vi "Get_SA_Spectrum_SubVI.vi"(8 "error in (no error)":errorcluster, 11 "IVI Refnum in":refnum<k15>) -> (0 "error out":errorcluster, 3 "IVI Refnum out":refnum<k15>)   [LabVIEW 2023]
uses:
  <instrlib>/Keysight XSAn/Keysight XSAn.lvlib
panel:
  out "Spectrum":cluster{"Frequency":dbl[], "Amplitude":dbl[]}
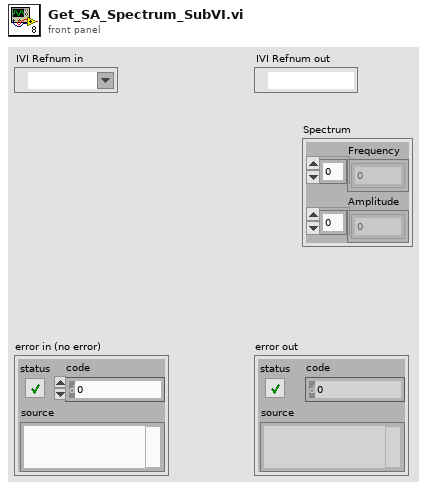
[diagram p1: front panel]
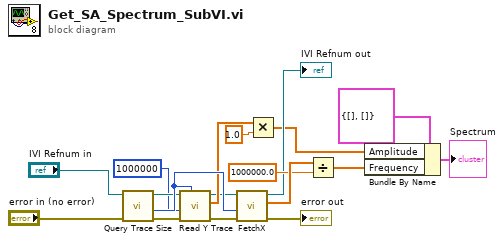
[diagram p0: block diagram]
diagram:
  n1 = call <instrlib>:"Query Trace Size.vi"("error in (no error)"="error in (no error)", "instrument handle"="IVI Refnum in") -> ("error out"=w16:errorcluster, "trace size"=w18:i32, "instrument handle out"=w17:refnum<k15>)  [unwired: 7 in]
  n2 = call <instrlib>:"Read Y Trace.vi"("array length"=w18, "error in (no error)"=w16, "maximum time"=1000000, "instrument handle"=w17) -> ("error out"=w9:errorcluster, "amplitude"=w13:dbl[], "instrument handle out"=w8:refnum<k15>)  [unwired: 4 in, 1 out]
  n3 = call "FetchX.vi"("error in (no error)"=w9, "ValBufferSize"=w18, "instrument handle"=w8) -> ("error out"=→"error out":errorcluster, "Val"=w10:dbl[], "instrument handle out"=→"IVI Refnum out":refnum<k15>)  [unwired: 5 in, 1 out]
  n4 = Multiply(x=w13, y=1.0) -> (x*y=w4:dbl[])
  n5 = Divide(x=w10, y=1000000.0) -> (x/y=w3:dbl[])
  n6 = Bundle By Name(cluster=cluster{"Frequency":dbl[], "Amplitude":dbl[]} {"Frequency"=[], "Amplitude"=[]} ("Spectrum"), "Amplitude"=w4, "Frequency"=w3) -> (→"Spectrum":cluster{"Frequency":dbl[], "Amplitude":dbl[]})
